vi "HAL camera get one frame old.vi"(2 "error in":errorcluster, 3 "New Image":T1, 4 "Camera Parameters (important)":T2={"Exposure Time (sec)"=0.0, "Readout Settings"={"Per-pixel gain compensation"=TRUE, "Readout speed"=TRUE}, "Image Size"={"Left"=0, "Top"=0, "Right"=1, "Bottom"=0, "Binning"=0}} {"Image Size"."Binning" items=["1 x 1"=1, "2 x 2"=2, "4 x 4"=4]; "Image Size"."Bottom" min=4 max=2048 step=4; "Image Size"."Right" min=4 max=2048 step=4; "Image Size"."Top" min=1 max=2048 step=4; "Image Size"."Left" min=1 max=2048 step=4; "Exposure Time (sec)" scale=0.001..10.0 scale format="%#_1g"}) -> (0 "error out":errorcluster, 1 "Image Out":T1)   [LabVIEW 2011]
uses:
  HAL camera parameters important.ctt
  orca readout settings.ctl
  image size.ctl
  <vilib>/vision/Image Controls.llb/IMAQ Image.ctl
  HAL Camera specifications globals.vi
panel:
  # "Camera: Hammamatsu Orca"
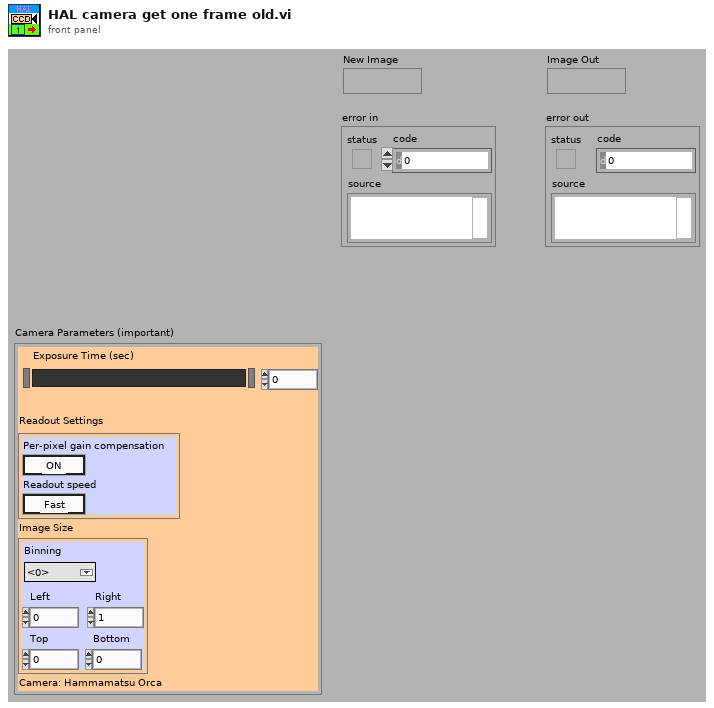
[diagram p1: front panel]
types:
  T1 = typedef "IMAQ Image.ctl" = refnum<image>
  T2 = typedef "HAL camera parameters important.ctt" = cluster{"Exposure Time (sec)":sgl, "Readout Settings":T3, "Image Size":T4}
  T3 = typedef "orca readout settings.ctl" = cluster{"Per-pixel gain compensation":bool, "Readout speed":bool}
  T4 = typedef "image size.ctl" = cluster{"Left":i32, "Top":i32, "Right":i32, "Bottom":i32, "Binning":u16}
  T5 = cluster{"width":u32, "height":u32, "datatype":u32}
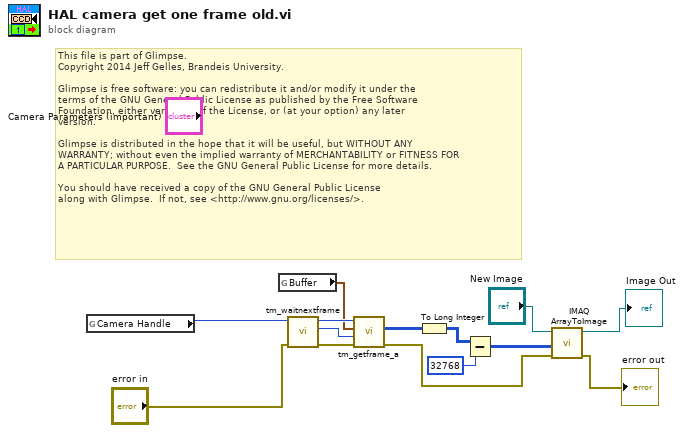
[diagram p0: block diagram]
diagram:
  # "This file is part of Glimpse. \nCopyright 2014 Jeff Gelles, Brandeis University.    \n\nGlimpse is free software: you can redistribute it and/or modify it under the \nterms of the GNU General Public License as published by the Free Software \nFoundation, either version 3 of the License, or (at your option) any later \nversion.\n\nGlimpse is distributed in the hope that it will be useful, but WITHOUT ANY \nWARRANTY; without even the implied warranty of MERCHANTABILITY or FITNESS FOR \nA PARTICULAR PURPOSE.  See the GNU General Public License for more details.\n\nYou should have received a copy of the GNU General Public License\nalong with Glimpse.  If not, see <http://www.gnu.org/licenses/>."
  n1 = global read "HAL Camera specifications globals.vi" "Camera Handle"() -> (w7:u32)
  n2 = global read "HAL Camera specifications globals.vi" "Buffer"() -> (w6:T5)
  n3 = call <userlib>:"tm_waitnextframe.vi"("error in (no error)"="error in", "Handle in"=w7) -> ("error out"=w13:errorcluster, "Frame Index"=w12:i32, "Handle out"=w14:u32)  [unwired: 6 in, 1 out]
  n4 = call <userlib>:"tm_getframe_a.vi"("error in (no error)"=w13, "Frame Index"=w12, "Buffer"=w6, "Handle in"=w14) -> ("error out"=w4:errorcluster, "Data 16"=w5:u16[][])  [unwired: 4 in, 2 out]
  n5 = To Long Integer(number=w5) -> (32bit integer=w11:i32[][])
  n6 = Subtract(x=w11, y=32768) -> (x-y=w10:i32[][])
  n7 = call "IMAQ ArrayToImage"("error in (no error)"=w4, "Image Pixels (I16)"=w10, "Image"="New Image") -> ("error out"=→"error out":errorcluster, "Image Out"=→"Image Out":T1)  [unwired: 3 in, 4 out]
